vi "Get Primary NIC IP Address and MAC.vi"(8 "error in":errorcluster, 11 "Session in":refnum<k21>) -> (0 "error out":errorcluster, 1 "IP Address Valid":bool, 2 "MAC Address":string, 3 "IP Address":string)   [LabVIEW 2015, in "SMI.lvlib" / "Device.lvclass"]
uses:
  Device.lvclass
  <vilib>/nisyscfg/Close (Hardware).vi
  <vilib>/nisyscfg/Close (System).vi
  <vilib>/nisyscfg/nisyscfg.lvlib
  <resource>/objmgr/niflexriosae.rc
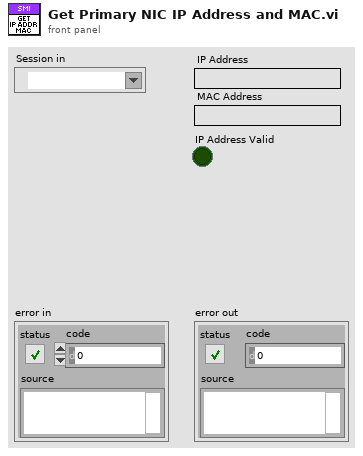
[diagram p1: front panel]
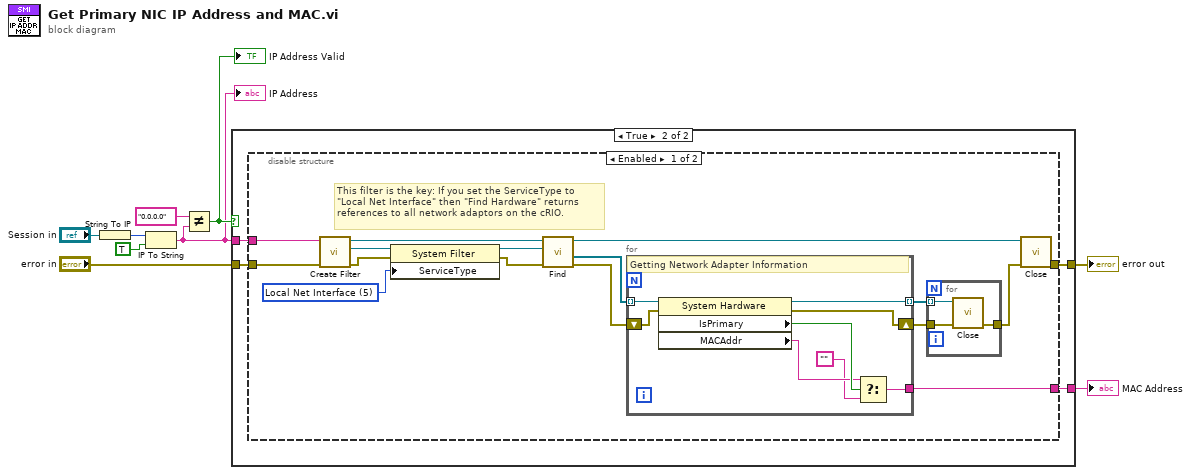
[diagram p0: block diagram]
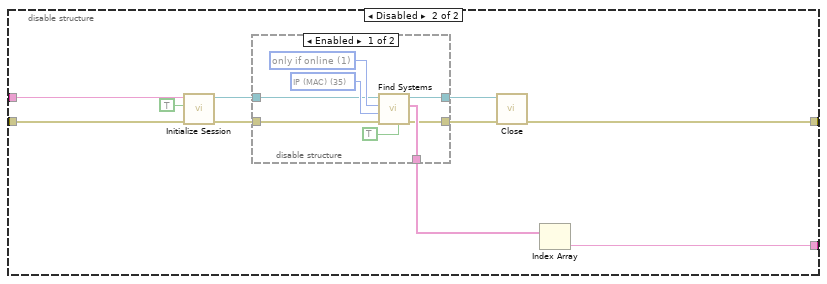
[diagram p3: hidden frame]
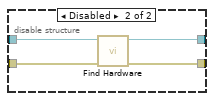
[diagram p4: hidden frame]
diagram:
  n1 = String To IP(1:"Session in") -> (0:w4:u32)
  n2 = IP To String(1:TRUE ("dot notation? (F)"), 2:w4) -> (0:w1:string)
  "IP Address" <- w1
  n3 = Not Equal?(x="0.0.0.0" ("y"), y=w1) -> (x != y?=w2:bool)
  "IP Address Valid" <- w2
  n4 = case shown="True" w2 {
    tunnel: "error in" -> [w10 w14]
    tunnel: [w10 w13] -> w8
    tunnel: [_ w12] -> w7
    tunnel: w1 -> [_ w11]
    frame False {
    }
    frame True {
      n5 = disable-structure shown="Enabled" {
        disable-tunnel: w14 -> [w21 w49]
        disable-tunnel: w11 -> [w20 w43]
        disable-tunnel: [w17 w44] -> w13
        disable-tunnel: [w15 w50] -> w12
        frame Enabled {
          w25 = u32 5 items=["NI Network Resource", "NI Real-Time", "NI System Configuration", "NI Web Interface", "Local System", "Local Net Interface", "Local Time Keeper", "Local Time Reference", "LXI Instrument"] ("Service Type")
          # "This filter is the key: If you set the ServiceType to\n\"Local Net Interface\" then \"Find Hardware\" returns\nreferences to all network adaptors on the cRIO."
          n6 = call <vilib>:"Create Filter.vi"("error in (no error)"=w21, "Session in"=w20) -> ("error out"=w28:errorcluster, "Filter out"=w24:refnum<k20>, "Session out"=w23:refnum<k21>)  [unwired: 7 in]
          n7 = property class="System Filter"(reference=w24, error in=w28, "ServiceType"=w25) -> (reference out=w26:refnum<k20>, error out=w27:errorcluster)
          n8 = call-poly <vilib>:"Find.vi"("error in (no error)"=w27, "Filter in"=w26, "Session in"=w23) -> ("error out"=w29:errorcluster, "Resources out"=w19:refnum<k20>[], "Session out"=w18:refnum<k21>)  [unwired: 5 in, 1 out]
          n9 = for {
            tunnel: w19 -> [w37] mode=indexing
            shift-right: [w35] -> w30
            shift-left: w29 -> [w38]
            tunnel: [w36] -> w22 mode=indexing
            tunnel: [w32] -> w15
            # "Getting Network Adapter Information"
            n10 = property class="System Hardware"(reference=w37, error in=w38) -> (reference out=w36:refnum<k20>, error out=w35:errorcluster, "IsPrimary"=w34:bool, "MACAddr"=w33:string)
            n11 = Select(t=w33, s=w34, f="") -> (s? t:f=w32:string)
          }
          n12 = for {
            tunnel: [w41] -> w16
            tunnel: w30 -> [w40]
            tunnel: w22 -> [w39] mode=indexing
            n13 = call-poly <vilib>:"Close.vi"("error in (no error)"=w40, "Resource in"=w39) -> ("error out"=w41:errorcluster)  [unwired: 9 in]
          }
          n14 = call-poly <vilib>:"Close.vi"("error in (no error)"=w16, "Session in"=w18) -> ("error out"=w17:errorcluster)  [unwired: 9 in]
        }
        frame Disabled {
          n15 = call <vilib>:"Initialize Session.vi"("error in (no error)"=w49, "Force Property Refresh (T)"=TRUE, "Target (localhost)"=w43) -> ("error out"=w48:errorcluster, "Session out"=w47:refnum<k21>)  [unwired: 7 in]
          n16 = disable-structure shown="Enabled" {
            disable-tunnel: [w57 _] -> w51
            disable-tunnel: w48 -> [w56 w63]
            disable-tunnel: w47 -> [w55 w61]
            disable-tunnel: [w54 w62] -> w45
            disable-tunnel: [w53 w60] -> w42
            frame Enabled {
              w58 = u32 35 items=["Hostname"=16, "Hostname (IP)"=18, "Hostname (MAC)"=19, "IP"=32, "IP (Hostname)"=33, "IP (MAC)"=35, "MAC"=48, "MAC (Hostname)"=49, "MAC (IP)"=50] ("Output (Hostname and IP)")
              w59 = u32 1 items=["none"=0, "only if online"=1, "all"=3] ("Include Cached Results (all)")
              n17 = call <vilib>:"Find Systems.vi"("Only Installable Systems (F)"=TRUE, "error in (no error)"=w56, "Output (Hostname and IP)"=w58, "Include Cached Results (all)"=w59, "Session in (localhost)"=w55) -> ("error out"=w54:errorcluster, "Detected Systems"=w57:string[], "Session out"=w53:refnum<k21>)  [unwired: 4 in]
            }
            frame Disabled {
              n18 = call <vilib>:"Find Hardware.vi"("error in (no error)"=w63, "Session in"=w61) -> ("error out"=w62:errorcluster, "Session out"=w60:refnum<k21>)  [unwired: 6 in, 2 out]
            }
          }
          n19 = call-poly <vilib>:"Close.vi"("error in (no error)"=w45, "Session in"=w42) -> ("error out"=w44:errorcluster)  [unwired: 9 in]
          n20 = Index Array(array=w51) -> (element=w50:string)  [unwired: 1 in]
        }
      }
    }
  }
  "error out" <- w8
  "MAC Address" <- w7
